vi "Status FGV.vi"(7 "Operation":enum16{"GET", "SET"}(ring), 8 "Error In":errorcluster, 11 "Red Edge Status In":T1) -> (0 "Error Out":errorcluster, 3 "Red Edge Status Out":T1)   [LabVIEW 2014]
uses:
  Controls/RedEdge Status.ctl
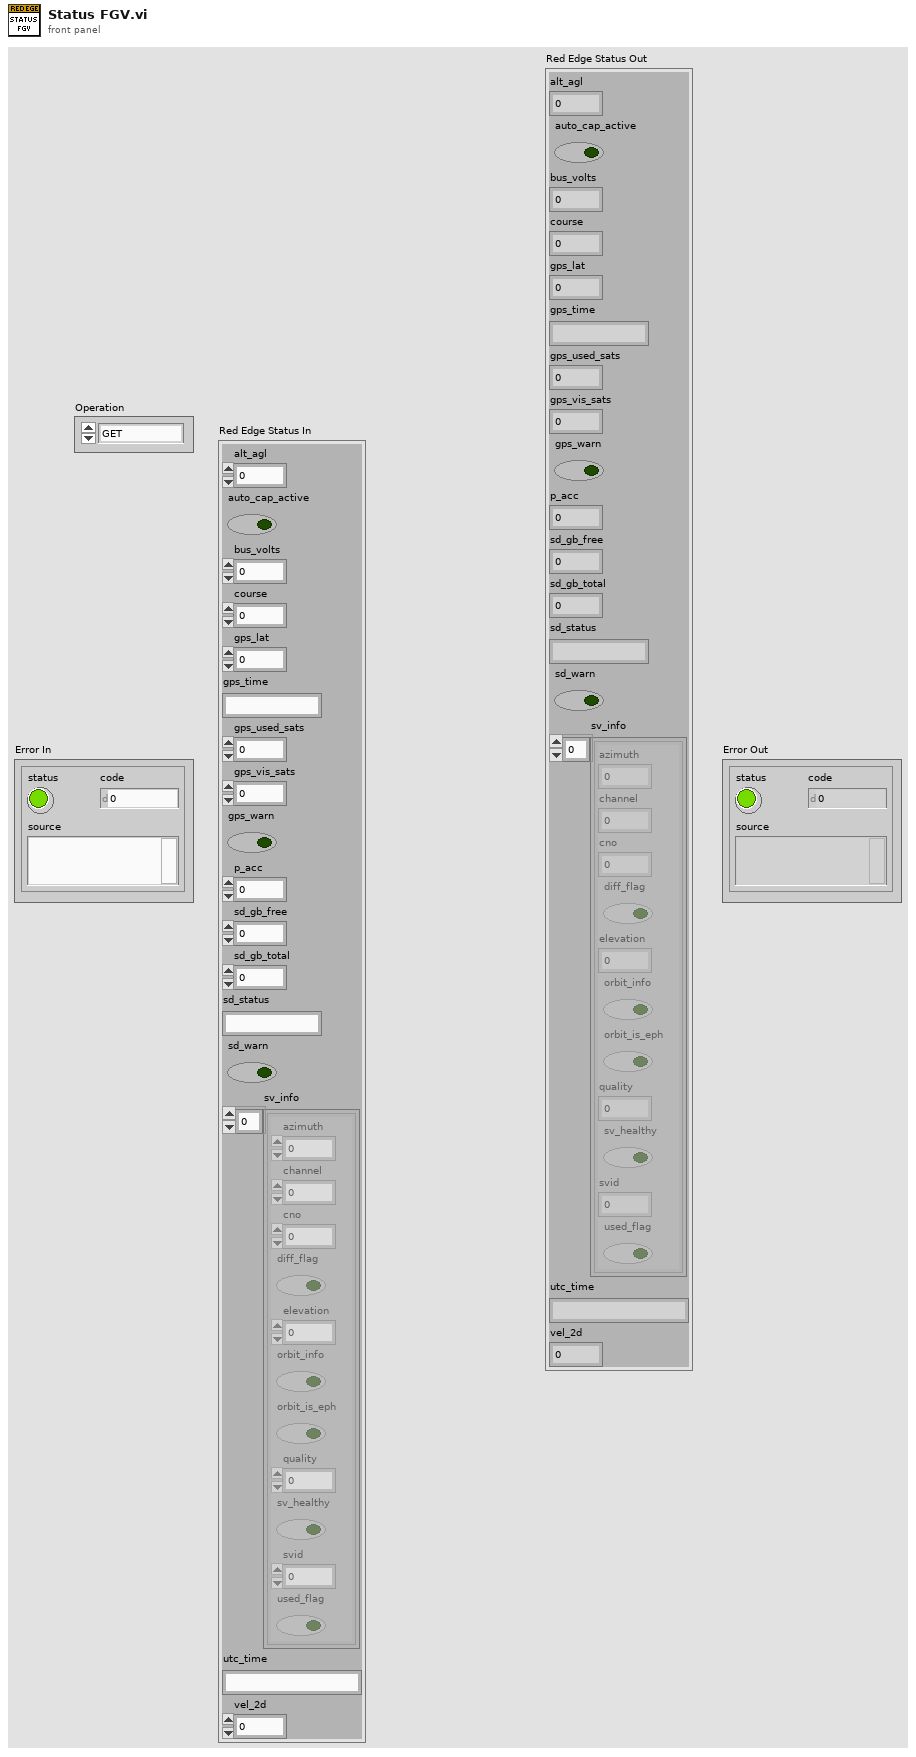
[diagram p1: front panel]
types:
  T1 = typedef "RedEdge Status.ctl" = cluster{"alt_agl":dbl, "auto_cap_active":bool, "bus_volts":i32, "course":i32, "gps_lat":dbl, "gps_time":string, "gps_used_sats":i32, "gps_vis_sats":i32, "gps_warn":bool, "p_acc":i32, "sd_gb_free":i32, "sd_gb_total":i32, "sd_status":string, "sd_warn":bool, "sv_info":cluster{"azimuth":i32, "channel":i32, "cno":i32, "diff_flag":bool, "elevation":i32, "orbit_info":bool, "orbit_is_eph":bool, "quality":i32, "sv_healthy":bool, "svid":i32, "used_flag":bool}[], "utc_time":string, "vel_2d":i32}
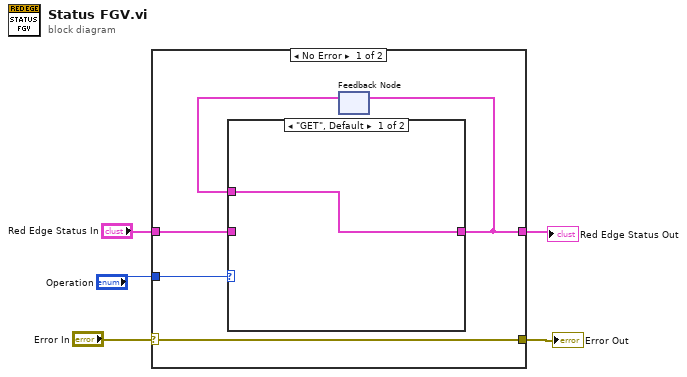
[diagram p0: block diagram]
diagram:
  n1 = case shown="No Error" "Error In" {
    selector: "Error In" -> [w6 w14]
    tunnel: "Operation" -> [w10 _]
    tunnel: "Red Edge Status In" -> [w9 w13]
    tunnel: [w8 w13] -> w3
    tunnel: [w6 w14] -> w1
    frame No Error {
      n2 = feedback #1() -> (w7:T1)  [unwired: 1 in]
      n3 = case shown="\"GET\", Default" w10 {
        tunnel: [w11 w12] -> w8
        tunnel: w9 -> [_ w12]
        tunnel: w7 -> [w11 _]
        frame "GET", Default {
        }
        frame "SET" {
        }
      }
      n4 = feedback-in #1(w8) -> ()
    }
    frame Error {
    }
  }
  "Red Edge Status Out" <- w3
  "Error Out" <- w1
